vi "SC_schleife_JT.vi"   [LabVIEW 2019]
uses:
  Monitors/Utility/Monitor Communication/LS370/LS370-Control.ctl
  Global/Global Variables/global.vi
  Monitors/Utility/Monitor Communication/sub-vis/LS370_Open_Queue.vi
  Instrument_Setup.vi
  Global/Global Variables/Data_Display_global.vi
types:
  T1 = typedef "LS370-Control.ctl" = cluster{"Disable Heater":bool, "Activate Tsweep":bool, "Update Lakeshores":bool, "Setpoint - Manual":dbl, "Rate (K/min)":dbl, "Sorb Power (mW)":dbl, "Still Power (mW)":dbl, "Sorb Heater":bool, "Still Heater":bool, "Set Temperature Sweep Main":bool}
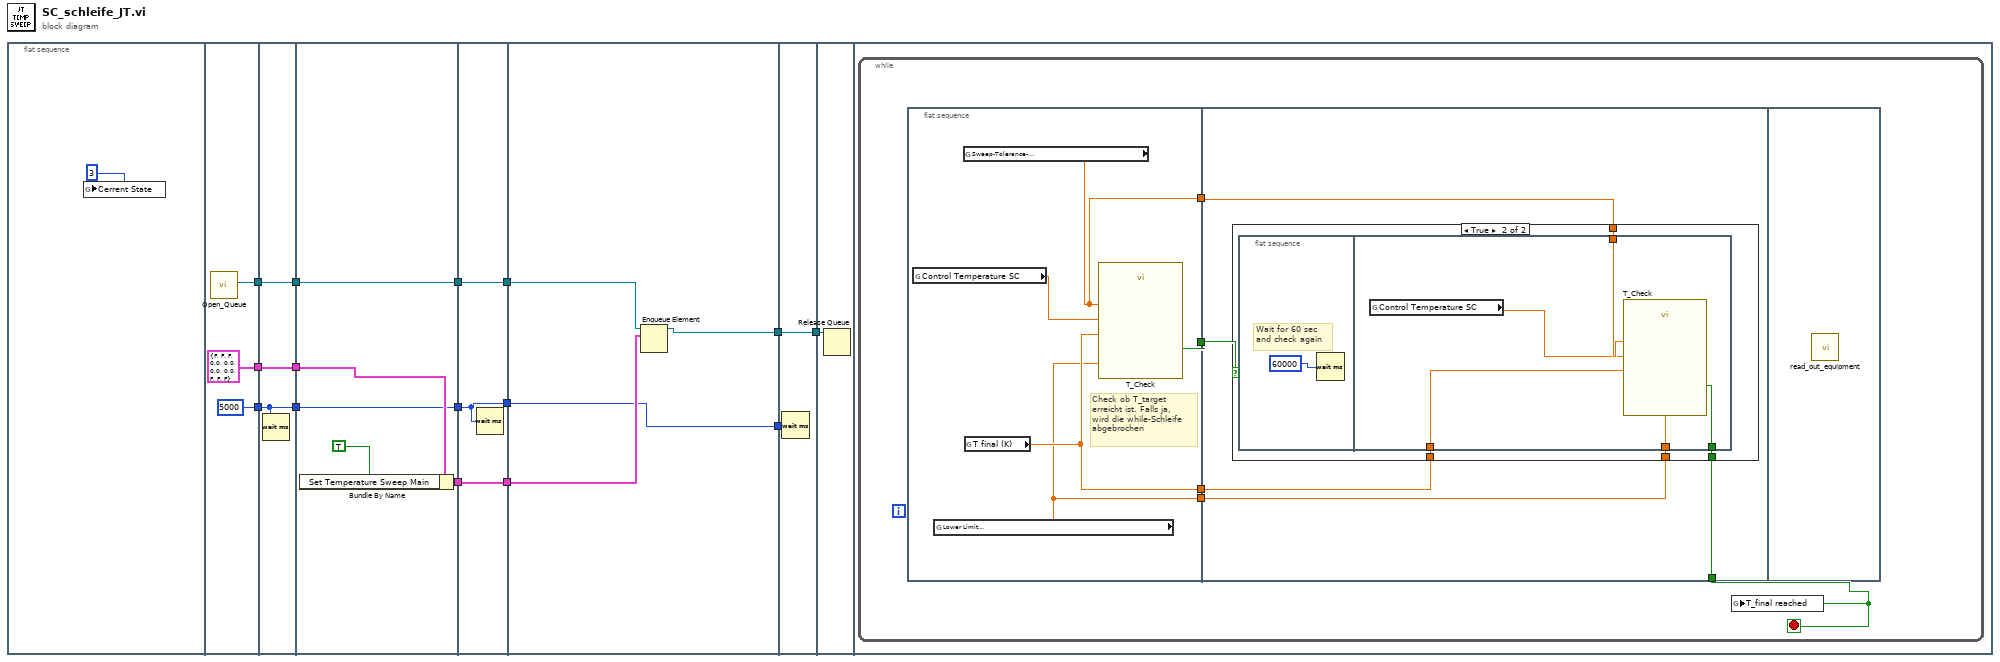
[diagram p0: block diagram]
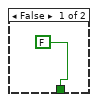
[diagram p2: hidden frame]
diagram:
  n1 = flat-sequence {
    tunnel: [w19] -> w15
    tunnel: [T1 {"Disable Heater"=FALSE, "Activate Tsweep"=FALSE, "Update Lakeshores"=FALSE, "Setpoint - Manual"=0.0, "Rate (K/min)"=0.0, "Sorb Power (mW)"=0.0, "Still Power (mW)"=0.0, "Sorb Heater"=FALSE, "Still Heater"=FALSE, "Set Temperature Sweep Main"=FALSE} ("JT-Cluster")] -> w13
    tunnel: [5000] -> w5
    tunnel: w15 -> [w22]
    tunnel: [w22] -> w14
    tunnel: w13 -> [w21]
    tunnel: [w21] -> w12
    tunnel: [w20] -> w6
    tunnel: w5 -> [w20]
    tunnel: w14 -> [w27]
    tunnel: [w27] -> w11
    tunnel: w12 -> [w26]
    tunnel: [w24] -> w9
    tunnel: [w23] -> w7
    tunnel: w6 -> [w23]
    tunnel: w11 -> [w30]
    tunnel: [w30] -> w10
    tunnel: w9 -> [w29]
    tunnel: [w29] -> w8
    tunnel: w7 -> [w28]
    tunnel: [w28] -> w2
    tunnel: w10 -> [w34]
    tunnel: w8 -> [w33]
    tunnel: [w32] -> w4
    tunnel: w2 -> [w31]
    tunnel: [w31] -> w1
    tunnel: w4 -> [w36]
    tunnel: [w36] -> w3
    tunnel: w1 -> [w35]
    tunnel: w3 -> [w37]
    frame #0 {
      n2 = global write "global.vi" "Cerrent State"(3) -> ()
    }
    frame #1 {
      n3 = call-poly "Open_Queue.vi"() -> ("queue out"=w19:refnum<queue>)  [unwired: 10 in, 1 out]
    }
    frame #2 {
      n4 = Wait (ms)(milliseconds to wait=w20) -> ()  [unwired: 1 out]
    }
    frame #3 {
      n5 = Bundle By Name(cluster=w26, "Set Temperature Sweep Main"=TRUE) -> (w24:T1)
    }
    frame #4 {
      n6 = Wait (ms)(milliseconds to wait=w28) -> ()  [unwired: 1 out]
    }
    frame #5 {
      n7 = Enqueue Element(queue=w34, element=w33) -> (queue out=w32:refnum<queue>)  [unwired: 2 in, 2 out]
    }
    frame #6 {
      n8 = Wait (ms)(milliseconds to wait=w35) -> ()  [unwired: 1 out]
    }
    frame #7 {
      n9 = Release Queue(queue=w37) -> ()  [unwired: 2 in, 3 out]
    }
    frame #8 {
      n10 = while {
        stop <- w39 stop-if-true
        n11 = flat-sequence {
          tunnel: [w47] -> w42
          tunnel: [w45] -> w41
          tunnel: [w46] -> w40
          tunnel: [w43] -> w38
          tunnel: w42 -> [w52]
          tunnel: w41 -> [w51]
          tunnel: w40 -> [w50]
          tunnel: [w49] -> w39
          tunnel: w38 -> [w48]
          frame #0 {
            # "Check ob T_target\nerreicht ist. Falls ja,\nwird die while-Schleife\nabgebrochen"
            n12 = global read "Data_Display_global.vi" "Control Temperature SC"() -> (w44:dbl)
            n13 = global read "Instrument_Setup.vi" "Lower Limit\nSweep-Tolerance-\nTemperature (K)"() -> (w43:dbl)
            n14 = global read "Instrument_Setup.vi" "Sweep-Tolerance-\nTemperature (%)"() -> (w46:dbl)
            n15 = global read "global.vi" "T final (K)"() -> (w45:dbl)
            n16 = call "T_Check.vi"("Lower Limit Sweep\nTolerance (K)"=w43, "T_target (K)"=w45, "Sweep\nTolerance %"=w46, "T_in"=w44) -> ("= T target"=w47:bool)
          }
          frame #1 {
            n17 = case shown="True" w52 {
              tunnel: w51 -> [_ w57]
              tunnel: w50 -> [_ w56]
              tunnel: [FALSE w55] -> w49
              tunnel: w48 -> [_ w54]
              frame False {
              }
              frame True {
                n18 = flat-sequence {
                  tunnel: w57 -> [w63]
                  tunnel: w56 -> [w62]
                  tunnel: [w61] -> w55
                  tunnel: w54 -> [w59]
                  frame #0 {
                    # "Wait for 60 sec\nand check again"
                    n19 = Wait (ms)(milliseconds to wait=60000) -> ()  [unwired: 1 out]
                  }
                  frame #1 {
                    n20 = global read "Data_Display_global.vi" "Control Temperature SC"() -> (w60:dbl)
                    n21 = call "T_Check.vi"("Lower Limit Sweep\nTolerance (K)"=w59, "T_target (K)"=w63, "Sweep\nTolerance %"=w62, "T_in"=w60) -> ("= T target"=w61:bool)
                  }
                }
              }
            }
          }
          frame #2 {
            n22 = call "read_out_equipment.vi"() -> ()  [unwired: 1 in]
          }
        }
        n23 = global write "Data_Display_global.vi" "T_final reached"(w39) -> ()
      }
    }
  }
